vi "Post Event.vi"(3 "error in (no error)":errorcluster, 4 "Event In":T1, 5 "Database.lvlib:Data Store.lvclass":refnum<class "Data Store.lvclass">) -> (0 "error out":errorcluster, 2 "Database.lvlib:Data Store.lvclass 2":refnum<class "Data Store.lvclass">)   [LabVIEW 2012, in "Database.lvlib" / "Data Store.lvclass"]
uses:
  Data Store.lvclass
  Dust Event.ctl
  Data Store.lvclass/Data Store.ctl
  <vilib>/addons/database/NI_Database_API.lvlib
  Database.lvlib
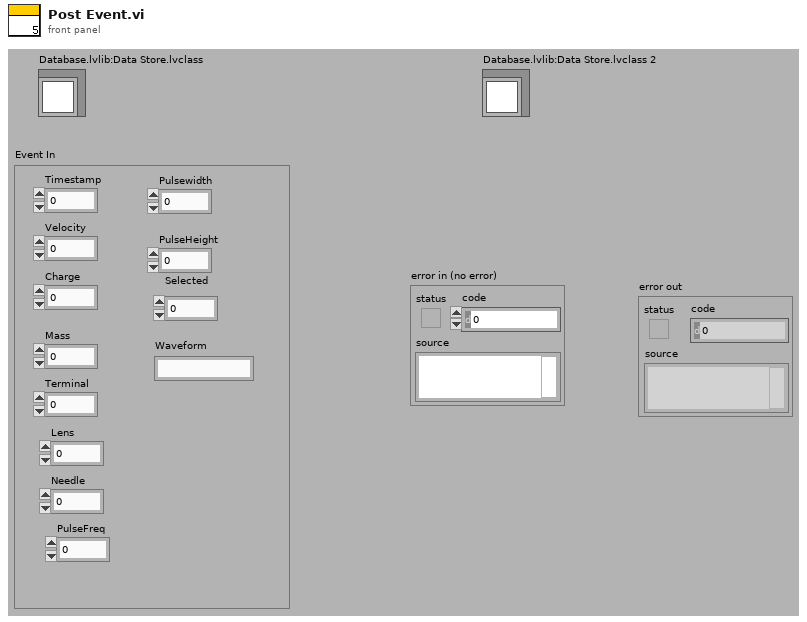
[diagram p1: front panel]
types:
  T1 = typedef "Database.lvlib/Dust Event.ctl" = cluster{"Timestamp":u64, "Velocity":sgl, "Charge":sgl, "Mass":sgl, "Terminal":sgl, "Lens":sgl, "Needle":sgl, "PulseFreq":sgl, "Pulsewidth":dbl, "PulseHeight":sgl, "Selected":i8, "Waveform":string}
  T2 = typedef "NI_Database_API.lvlib/Conn ObjectReference.ctl" = refnum<k1>
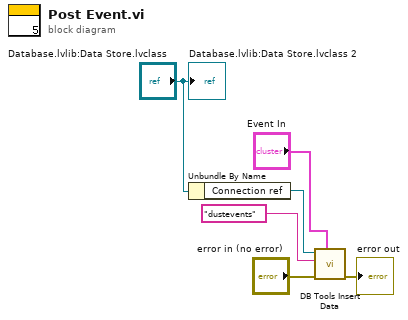
[diagram p0: block diagram]
diagram:
  n1 = Unbundle By Name("Database.lvlib:Data Store.lvclass") -> ("Connection ref"=w5:T2)
  n2 = call <vilib>:"DB Tools Insert Data.vi"("data"="Event In", "error in (no error)"="error in (no error)", "table"="dustevents", "connection reference"=w5) -> ("error out"=→"error out":errorcluster)  [unwired: 6 in, 1 out]
  "Database.lvlib:Data Store.lvclass 2" <- "Database.lvlib:Data Store.lvclass"
